vi "ASDA-A2_Get DI Status.vi"(8 "error in":errorcluster, 11 "Buffer Data In":T2) -> (0 "error out":errorcluster, 2 "DI Status":T1, 3 "Buffer Data Out":T2)   [LabVIEW 2016]
uses:
  Data Def/ASDA-A2_Buffer Data.ctl
  Data Def/ASDA-A2_Read Register Data.ctl
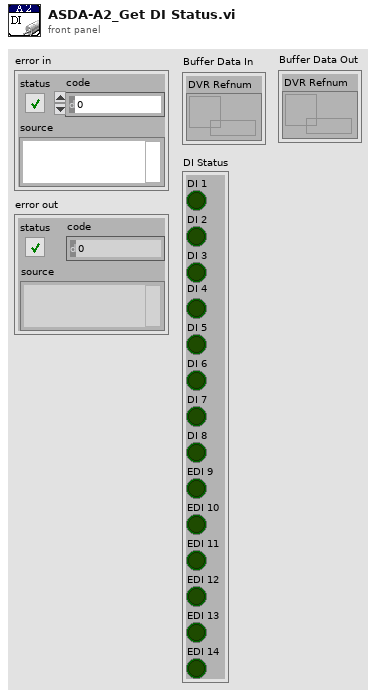
[diagram p1: front panel]
types:
  T1 = cluster{"DI 1":bool, "DI 2":bool, "DI 3":bool, "DI 4":bool, "DI 5":bool, "DI 6":bool, "DI 7":bool, "DI 8":bool, "EDI 9":bool, "EDI 10":bool, "EDI 11":bool, "EDI 12":bool, "EDI 13":bool, "EDI 14":bool}
  T2 = typedef "ASDA-A2_Buffer Data.ctl" = cluster{"DVR Refnum":refnum<data-value>}
  T3 = typedef "ASDA-A2_Read Register Data.ctl" = cluster{"Address":u16, "Count":u16, "Page":string, "Description":string}
  T4 = cluster{"Boolean array[0]":bool, "Boolean array[1]":bool, "Boolean array[2]":bool, "Boolean array[3]":bool, "Boolean array[4]":bool, "Boolean array[5]":bool, "Boolean array[6]":bool, "Boolean array[7]":bool, "Boolean array[8]":bool, "Boolean array[9]":bool, "Boolean array[10]":bool, "Boolean array[11]":bool, "Boolean array[12]":bool, "Boolean array[13]":bool}
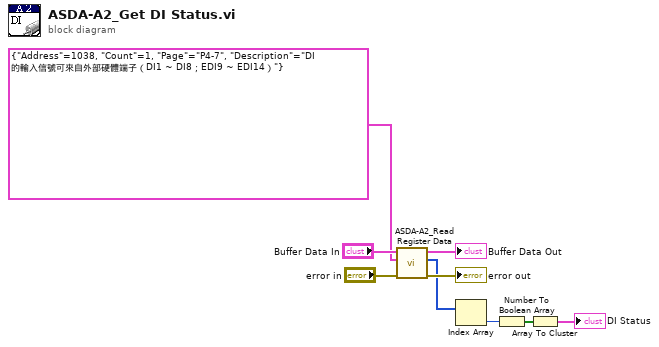
[diagram p0: block diagram]
diagram:
  n1 = call "ASDA-A2_Read Register Data.vi"("error in"="error in", "Read Register Data"=T3 {"Address"=1038, "Count"=1, "Page"="P4-7", "Description"="DI 的輸入信號可來自外部硬體端子（DI1 ~ DI8；EDI9 ~ EDI14）"}, "Buffer Data In"="Buffer Data In") -> ("error out"=→"error out":errorcluster, "Data"=w4:u16[], "Buffer Data Out"=→"Buffer Data Out":T2)  [unwired: 6 in]
  n2 = Index Array(array=w4) -> (element=w2:u16)  [unwired: 1 in]
  n3 = Number To Boolean Array(number=w2) -> (Boolean array=w3:bool[])
  n4 = Array To Cluster(array=w3) -> (cluster=→"DI Status":T4)
